vi "Temperature_System.vi"() -> ()   [LabVIEW 2022 SP3]
uses:
  <vilib>/Analysis/NI_AALBase.lvlib
panel:
  in  "Return to Menu":bool
  out "Waveform Graph":dbl[](graph)
  in  "Return to Menu":bool
  out "Histogram":T1(graph)
  in  "?":bool
  in  "Chart Type":u16(ring) items=["Histogram", "Waveform"]
  out "RandCel":dbl[](array[numeric])
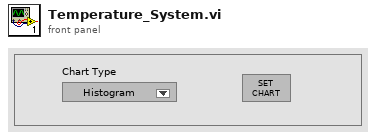
[diagram p1: front panel]
types:
  T1 = cluster{"X Values":dbl[], "Histogram: h(x)":i32[]}
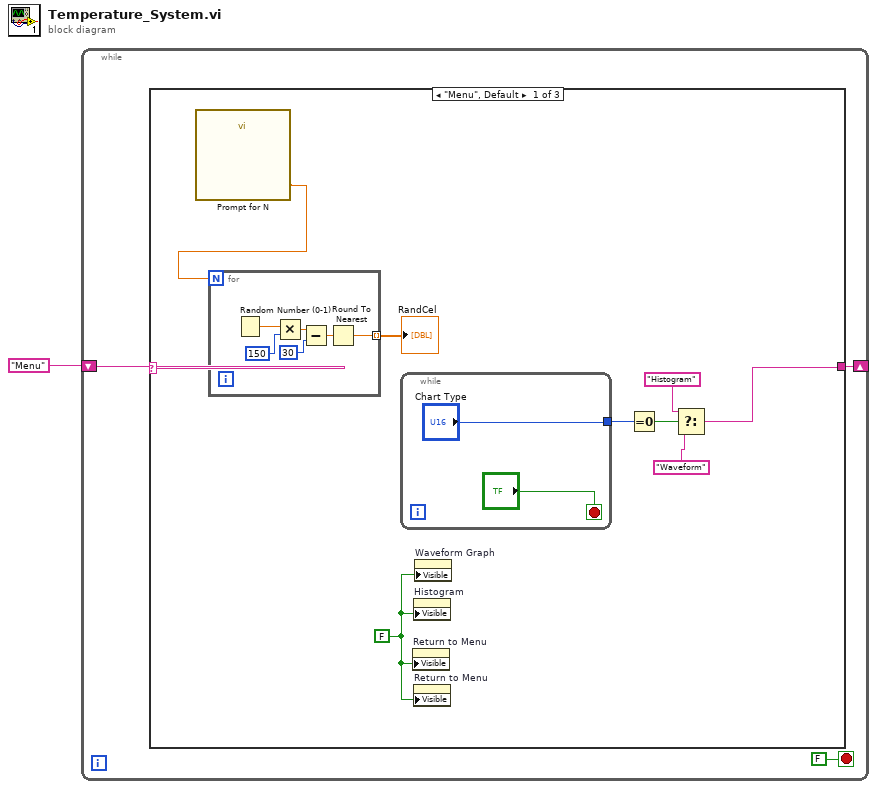
[diagram p0: block diagram]
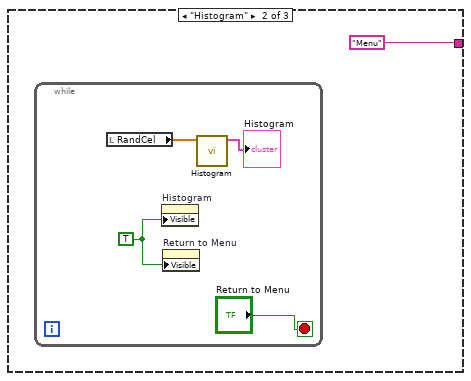
[diagram p2: hidden frame]
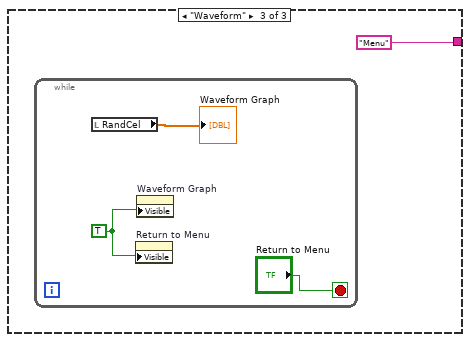
[diagram p3: hidden frame]
diagram:
  n1 = while {
    shift-right: [w3] -> _
    shift-left: "Menu" -> [w4]
    stop <- FALSE stop-if-true
    n2 = case shown="\"Menu\", Default" w4 {
      tunnel: [w8 "Menu" "Menu"] -> w3
      frame "Menu", Default {
        w7 = FALSE
        n3 = call "Prompt for N"() -> ("N"=w5:dbl)  [unwired: 17 in, 2 out]
        n4 = for {
          N: w5 -> [_]
          tunnel: [w13] -> w6 mode=indexing
          n5 = Random Number (0-1)() -> (number: 0 to 1=w17:dbl)
          n6 = Multiply(x=w17, y=150) -> (x*y=w18:dbl)
          n7 = Subtract(x=w18, y=30) -> (x-y=w14:dbl)
          n8 = Round To Nearest(number=w14) -> (nearest integer value=w13:dbl)
        }
        "RandCel" <- w6
        n9 = while {
          tunnel: ["Chart Type"] -> w12
          stop <- "?" stop-if-true
        }
        n10 = property on="Return to Menu" class="Bool"("Visible"=w7) -> ()  [unwired: 2 in, 2 out]
        n11 = property on="Histogram" class="XYGraph (strict)"("Visible"=w7) -> ()  [unwired: 2 in, 2 out]
        n12 = property on="Return to Menu" class="Bool"("Visible"=w7) -> ()  [unwired: 2 in, 2 out]
        n13 = property on="Waveform Graph" class="WFGraph (strict)"("Visible"=w7) -> ()  [unwired: 2 in, 2 out]
        n14 = Equal To 0?(x=w12) -> (x = 0?=w11:bool)
        n15 = Select(t="Histogram", s=w11, f="Waveform") -> (s? t:f=w8:string)
      }
      frame "Histogram" {
        n16 = while {
          stop <- "Return to Menu" stop-if-true
          w22 = TRUE
          n17 = local read "RandCel"() -> (w25:dbl[])
          n18 = property on="Histogram" class="XYGraph (strict)"("Visible"=w22) -> ()  [unwired: 2 in, 2 out]
          n19 = property on="Return to Menu" class="Bool"("Visible"=w22) -> ()  [unwired: 2 in, 2 out]
          n20 = call <vilib>:"Histogram.vi"("X"=w25) -> ("Histogram Graph"=→"Histogram":T1)  [unwired: 7 in, 3 out]
        }
      }
      frame "Waveform" {
        n21 = while {
          stop <- "Return to Menu" stop-if-true
          w28 = TRUE
          n22 = local read "RandCel"() -> (→"Waveform Graph":dbl[])
          n23 = property on="Return to Menu" class="Bool"("Visible"=w28) -> ()  [unwired: 2 in, 2 out]
          n24 = property on="Waveform Graph" class="WFGraph (strict)"("Visible"=w28) -> ()  [unwired: 2 in, 2 out]
        }
      }
    }
  }
